vi "config.write.vi"(8 "error in (no error)":errorcluster, 11 "paths":T1) -> (0 "error out":errorcluster)   [LabVIEW 2024, in "Shared.lvlib"]
uses:
  Shared.lvlib
  paths--cluster.ctl
  <vilib>/addons/_JKI.lib/Serialization/JSON/JKI JSON Serialization.lvlib
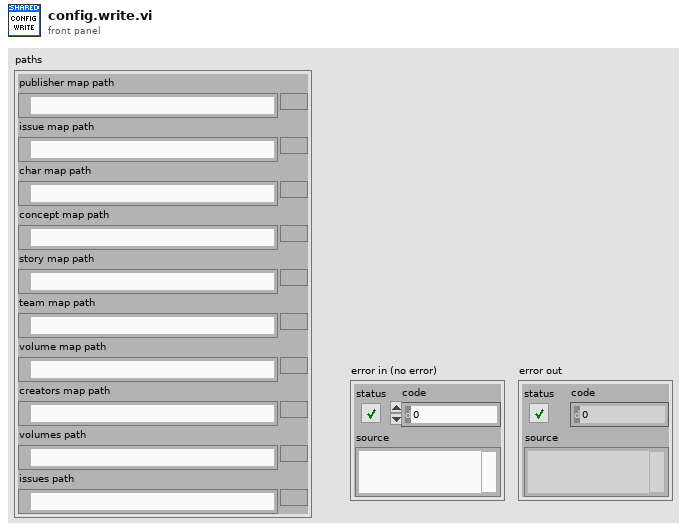
[diagram p1: front panel]
types:
  T1 = typedef "Shared.lvlib/paths--cluster.ctl" = cluster{"publisher map path":path, "issue map path":path, "char map path":path, "concept map path":path, "story map path":path, "team map path":path, "volume map path":path, "creators map path":path, "volumes path":path, "issues path":path}
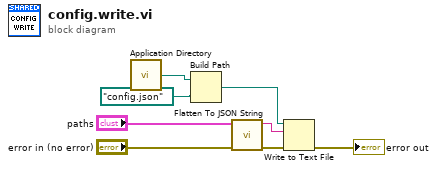
[diagram p0: block diagram]
diagram:
  n1 = call <vilib>:"Application Directory.vi"() -> ("Application Directory"=w8:path)
  n2 = Build Path(base path=w8, name or relative path=path "config.json") -> (appended path=w2:path)
  n3 = call <vilib>:"Flatten To JSON String.vi"("error in"="error in (no error)", "Variant"="paths") -> ("error out"=w4:errorcluster, "JSON String"=w3:string)  [unwired: 8 in]
  n4 = Write to Text File(file (use dialog)=w2, text=w3, error in=w4) -> (error out=→"error out":errorcluster)  [unwired: 1 in, 2 out]
